vi "ListenForClient.vi"(8 "error in (no error)":errorcluster, 11 "Server in":refnum<class "Server.lvclass">) -> (0 "error out":errorcluster, 3 "Server out":refnum<class "Server.lvclass">)   [LabVIEW 2021, in "Server.lvlib" / "Server.lvclass"]
uses:
  Server.lvclass
  C:/Program Files/National Instruments/LabVIEW 2021/vi.lib/ActorFramework/Actor/Actor.lvclass
  <vilib>/NI/Actors/Network Endpoint Actors/Nested Endpoint/Nested Endpoint/Nested Endpoint.lvclass
  C:/Program Files/National Instruments/LabVIEW 2021/vi.lib/NI/Actors/Network Endpoint Actors/Network Endpoint/Network Endpoint/Network Endpoint.lvclass
  Server Messages/Connected Msg/Connected Msg.lvclass
  C:/Program Files/National Instruments/LabVIEW 2021/vi.lib/NI/Actors/Network Endpoint Actors/Nested Endpoint/Nested Endpoint Messages/Connected Msg/Connected Msg.lvclass
  Server.lvclass/Server.ctl
  <vilib>/NI/Actors/Network Endpoint Actors/Network Endpoint/Network Endpoint/Network Endpoint.lvclass/Network Endpoint.ctl
  <vilib>/NI/Actors/Network Endpoint Actors/Nested Endpoint/Nested Endpoint/Nested Endpoint.lvclass/Nested Endpoint.ctl
  <vilib>/NI/Actors/Network Endpoint Actors/Protocols/TCP Strategy/TCP Stream Listener/TCP Stream Listener.lvclass
  C:/Program Files/National Instruments/LabVIEW 2021/vi.lib/NI/Actors/Network Endpoint Actors/Abstract Classes/Message Stream/Message Stream.lvclass
  <vilib>/ActorFramework/Actor/Actor.lvclass
  <vilib>/NI/Actors/Network Endpoint Actors/Network Endpoint/Network Endpoint/Network Endpoint.lvclass
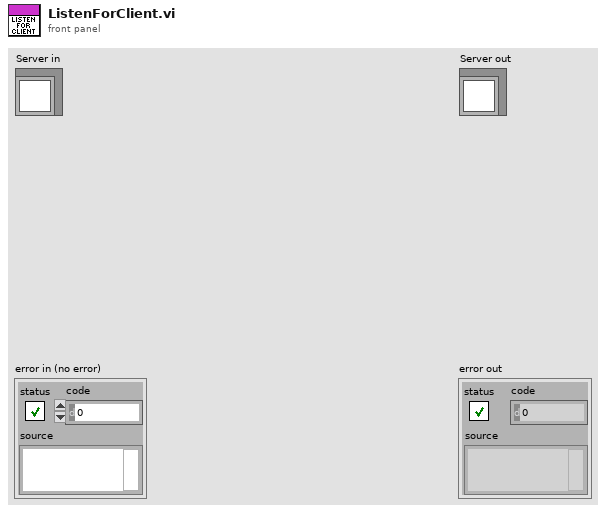
[diagram p1: front panel]
types:
  T1 = enum8{"Enabled", "Disabled", "Disabled and Grayed Out"}
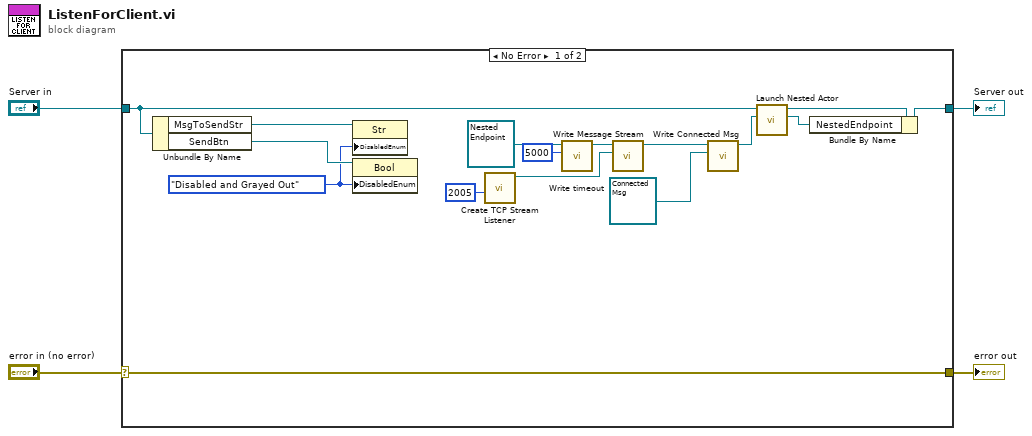
[diagram p0: block diagram]
diagram:
  n1 = case shown="No Error" "error in (no error)" {
    selector: "error in (no error)" -> [w20 w22]
    tunnel: [w20 w22] -> w3
    tunnel: [w12 w21] -> w1
    tunnel: "Server in" -> [w10 w21]
    frame No Error {
      w7 = T1."Disabled and Grayed Out" ("Disabled")
      n2 = Unbundle By Name(w10) -> ("MsgToSendStr"=w9:refnum<vi>, "SendBtn"=w8:refnum<vi>)
      n3 = property class="Str"(reference=w9, "DisabledEnum"=w7) -> ()  [unwired: 1 in, 2 out]
      n4 = property class="Bool"(reference=w8, "DisabledEnum"=w7) -> ()  [unwired: 1 in, 2 out]
      n5 = call <vilib>:"Create TCP Stream Listener.vi"("Local Port"=u16 2005) -> ("TCP Stream Listener"=w14:refnum<class "TCP Stream Listener.lvclass">)  [unwired: 10 in]
      n6 = call <vilib>:"Write timeout.vi"("timeout"=5000, "Network Endpoint in"=refnum<class "Nested Endpoint.lvclass"> refnum ("Nested Endpoint.lvlib:Nested Endpoint.lvclass")) -> ("Network Endpoint out"=w15:refnum<class "Nested Endpoint.lvclass">)  [unwired: 9 in]
      n7 = call <vilib>:"Write Message Stream.vi"("Message Stream"=w14, "Network Endpoint in"=w15) -> ("Network Endpoint out"=w13:refnum<class "Nested Endpoint.lvclass">)  [unwired: 9 in]
      n8 = call <vilib>:"Write Connected Msg.vi"("Nested Endpoint.lvlib:Connected Msg.lvclass"=refnum<class "Connected Msg.lvclass"> refnum ("Server.lvlib:Connected Msg.lvclass"), "Nested Endpoint in"=w13) -> ("Nested Endpoint out"=w6:refnum<class "Nested Endpoint.lvclass">)  [unwired: 9 in]
      n9 = call <vilib>:"Launch Nested Actor.vi"("Nested Actor"=w6, "Caller Actor in"=w10) -> ("Nested Actor's Enqueuer"=w11:refnum<class "Message Enqueuer.lvclass">, "Caller Actor out"=w19:refnum<class "Server.lvclass">)  [unwired: 7 in, 1 out]
      n10 = Bundle By Name(cluster=w19, "NestedEndpoint"=w11) -> (w12:refnum<class "Server.lvclass">)
    }
    frame Error {
    }
  }
  "error out" <- w3
  "Server out" <- w1
